vi "Read.vi"(8 "error in (no error)":errorcluster, 9 "timeout ms (5000)":i32=5000, 11 "WebSocket Connection in":refnum<k5>) -> (0 "error out":errorcluster, 1 "Opcode":T1=1 items=["Cont. Frame"=0, "Text"=1, "Binary"=2, "Ping"=9, "Pong"=10], 2 "Data":string, 3 "WebSocket Connection out":refnum<k5>, 4 "Finished?":bool)   [LabVIEW 2013, in "WebSockets.lvlib"]
doc: "Reads and decodes an incoming WebSockets message.\n\nOpcode: Opcode for the message.\nData: Contains the WebSockets payload\nFinished?: Determines whether the message is complete for fragmented messages. If false, must continue to read messages (continuation frames with opcode = 0) until Finished? is true."
uses:
  WebSockets.lvlib
  Opcodes.ctl
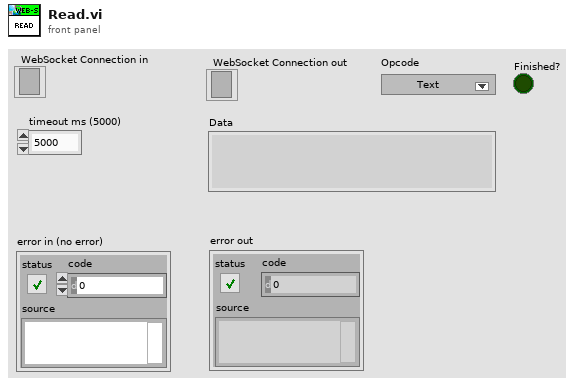
[diagram p1: front panel]
types:
  T1 = typedef "WebSockets.lvlib/Opcodes.ctl" = u8
  T2 = enum16{"big-endian, network order", "native, host order", "little-endian"}
  T3 = enum16{"Standard", "Buffered", "CRLF", "Immediate"}
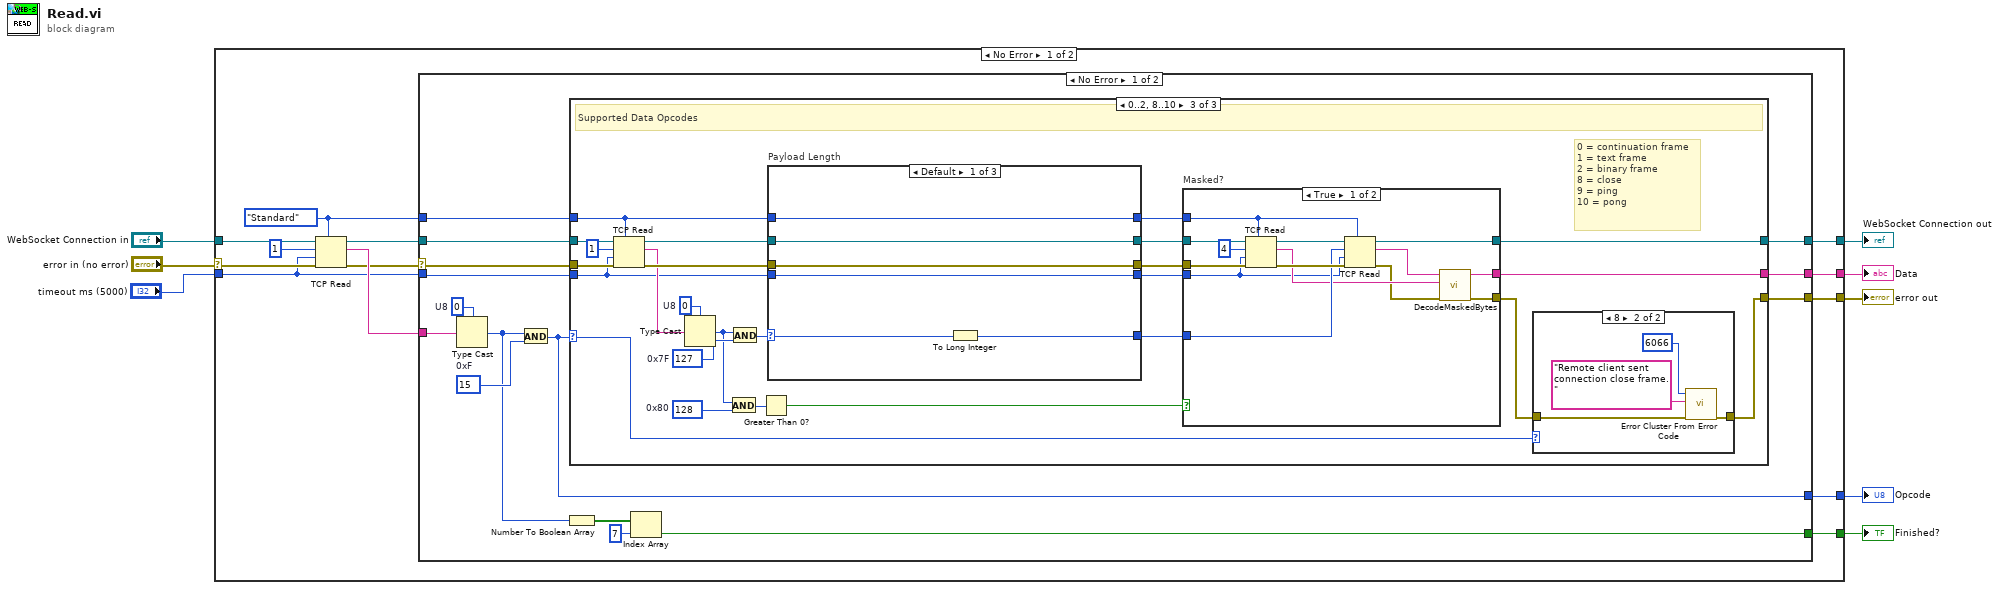
[diagram p0: block diagram]
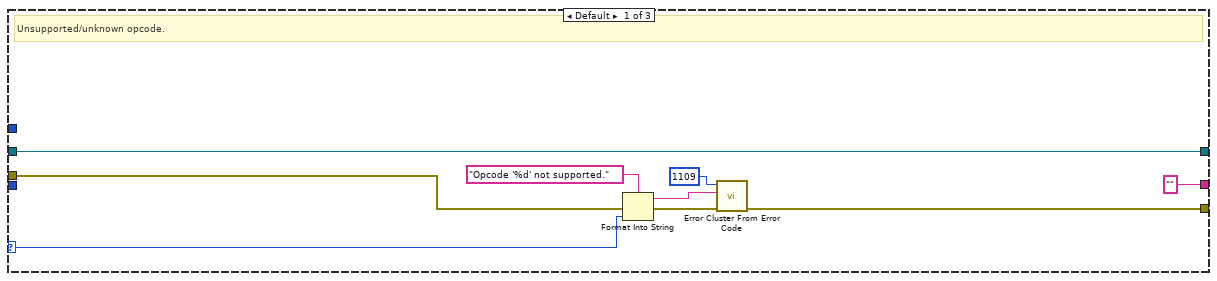
[diagram p2: hidden frame]
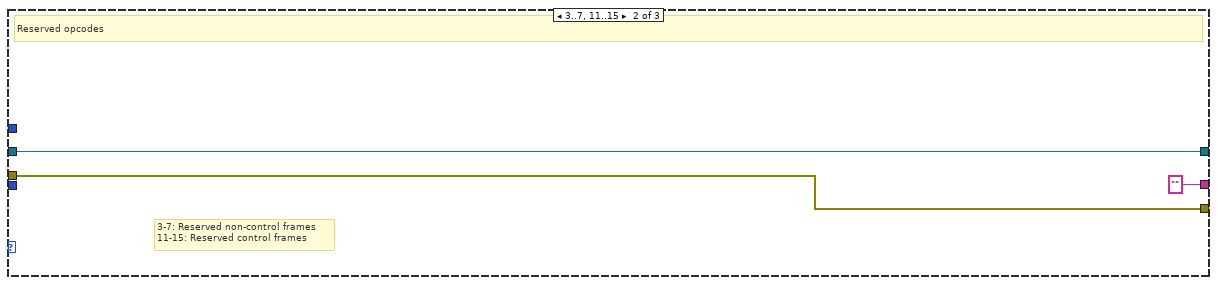
[diagram p3: hidden frame]
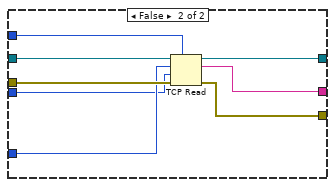
[diagram p5: hidden frame]
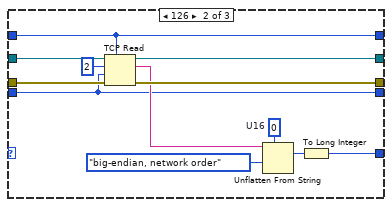
[diagram p6: hidden frame]
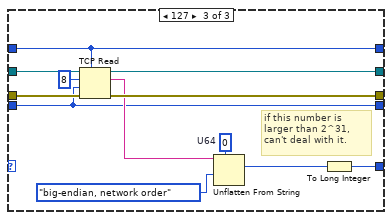
[diagram p7: hidden frame]
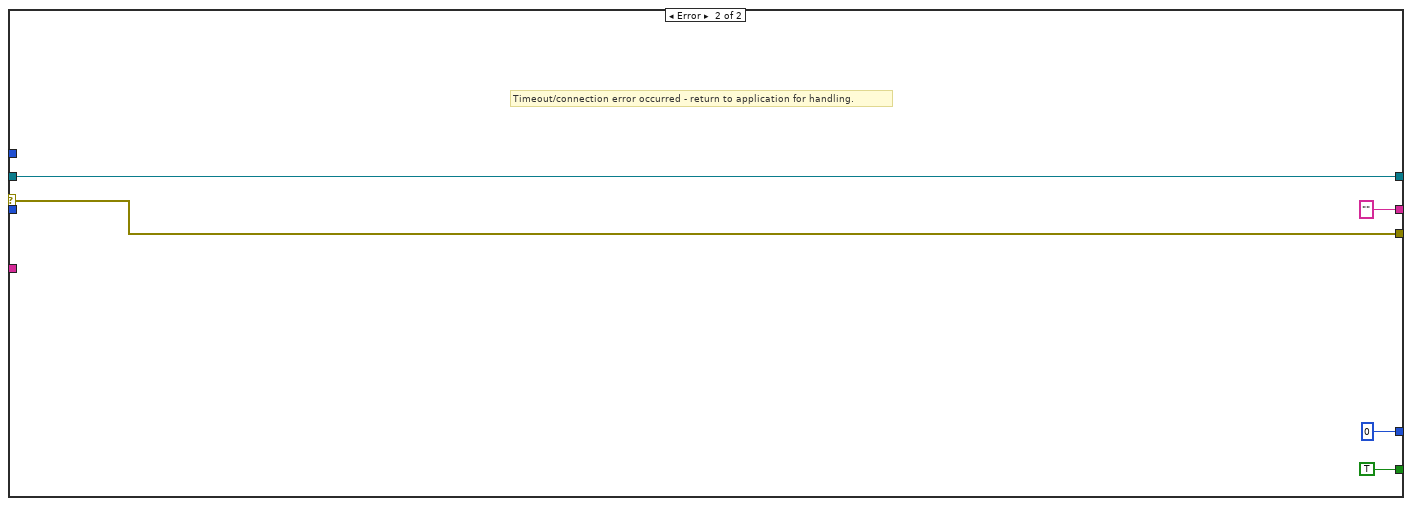
[diagram p8: hidden frame]
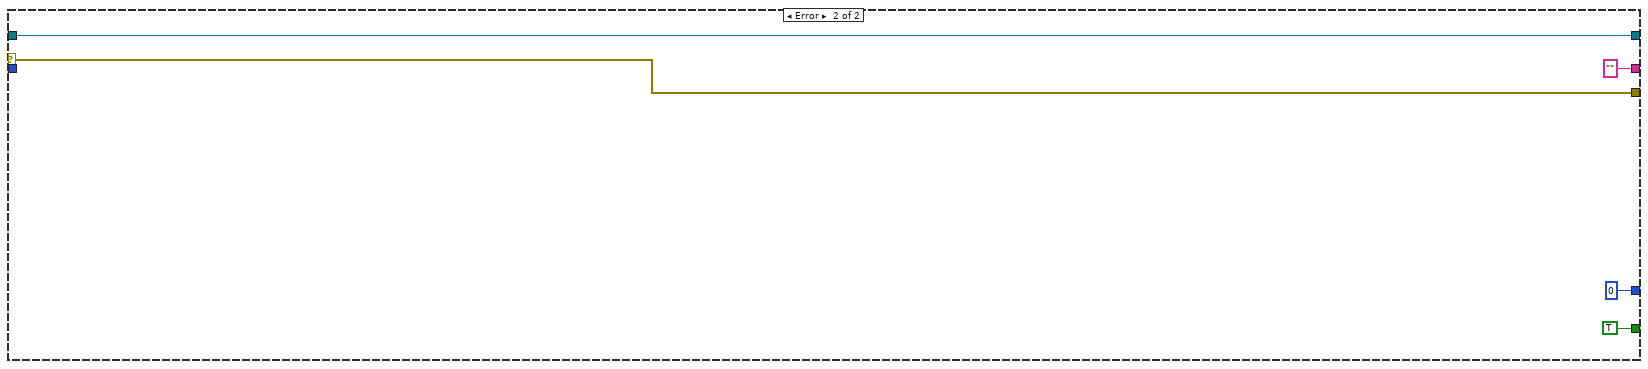
[diagram p9: hidden frame]
diagram:
  n1 = case shown="No Error" "error in (no error)" {
    selector: "error in (no error)" -> [w15 w140]
    tunnel: "WebSocket Connection in" -> [w21 w139]
    tunnel: [w16 w139] -> w7
    tunnel: [w14 "" ("data out")] -> w6
    tunnel: [w13 w140] -> w4
    tunnel: "timeout ms (5000)" -> [w9 _]
    tunnel: [w11 u8 0] -> w1
    tunnel: [w10 TRUE] -> w2
    frame No Error {
      w17 = T3."Standard" ("mode (standard)")
      n2 = TCP Read(connection ID=w21, bytes to read=1, error in (no error)=w15, 7:w17, 9:w9) -> (connection ID out=w18:refnum<k5>, data out=w19:string, error out=w12:errorcluster)
      n3 = case shown="No Error" w12 {
        selector: w12 -> [w31 w133]
        tunnel: w19 -> [w30 _]
        tunnel: w18 -> [w36 w135]
        tunnel: w17 -> [w35 _]
        tunnel: [w34 w135] -> w16
        tunnel: [w33 "" ("Decoded Data")] -> w14
        tunnel: [w32 w133] -> w13
        tunnel: [w27 u8 0] -> w11
        tunnel: [w24 TRUE] -> w10
        tunnel: w9 -> [w23 _]
        frame No Error {
          w28 = u8 15  # 0xF
          w29 = u8 0  # U8
          n4 = Type Cast(type=w29, x=w30) -> (*(type *) &x=w26:u8)
          n5 = And(x=w26, y=w28) -> (x .and. y?=w27:u8)
          n6 = Number To Boolean Array(number=w26) -> (Boolean array=w25:bool[])
          n7 = case shown="0..2, 8..10" w27 {
            selector: w27 -> [w38 _ w53]
            tunnel: w36 -> [w45 w47 w65]
            tunnel: w35 -> [_ _ w63]
            tunnel: [w45 w47 w73] -> w34
            tunnel: ["" ("Decoded Data") "" ("Decoded Data") w66] -> w33
            tunnel: [w43 w48 w51] -> w32
            tunnel: w31 -> [w42 w48 w61]
            tunnel: w23 -> [_ _ w49]
            frame Default {
              # "Unsupported/unknown opcode."
              n8 = Format Into String(format string="Opcode '%d' not supported.", error in=w42, w38) -> (resulting string=w40:string, error out=w41:errorcluster)  [unwired: 1 in]
              n9 = call <vilib>:"Error Cluster From Error Code.vi"("error in (no error)"=w41, "error message (\"\")"=w40, "error code (0)"=1109) -> ("error out"=w43:errorcluster)  [unwired: 6 in]
            }
            frame 3..7, 11..15 {
              # "3-7: Reserved non-control frames\n11-15: Reserved control frames"
              # "Reserved opcodes"
            }
            frame 0..2, 8..10 {
              w57 = u8 128  # 0x80
              w58 = u8 0  # U8
              w72 = u8 127  # 0x7F
              # "0 = continuation frame\n1 = text frame\n2 = binary frame\n8 = close\n9 = ping\n10 = pong"
              # "Supported Data Opcodes"
              n10 = TCP Read(connection ID=w65, bytes to read=1, error in (no error)=w61, 7:w63, 9:w49) -> (connection ID out=w64:refnum<k5>, data out=w59:string, error out=w60:errorcluster)
              n11 = Type Cast(type=w58, x=w59) -> (*(type *) &x=w56:u8)
              n12 = And(x=w56, y=w57) -> (x .and. y?=w55:u8)
              n13 = And(x=w56, y=w72) -> (x .and. y?=w71:u8)
              n14 = Greater Than 0?(x=w55) -> (x > 0?=w54:bool)
              n15 = case "Payload Length" shown="Default" w71 {
                selector: w71 -> [w105 _ _]
                tunnel: w64 -> [w106 w118 w129]
                tunnel: [w106 w117 w128] -> w70
                tunnel: w63 -> [w103 w115 w124]
                tunnel: [w104 w108 w127] -> w67
                tunnel: [w103 w115 w124] -> w69
                tunnel: [w102 w114 w126] -> w68
                tunnel: w60 -> [w102 w113 w125]
                tunnel: w49 -> [w101 w107 w119]
                tunnel: [w101 w107 w119] -> w50
                frame Default {
                  n16 = To Long Integer(number=w105) -> (32bit integer=w104:i32)
                }
                frame 126 {
                  w112 = u16 0  # U16
                  n17 = TCP Read(connection ID=w118, bytes to read=2, error in (no error)=w113, 7:w115, 9:w107) -> (connection ID out=w117:refnum<k5>, data out=w110:string, error out=w114:errorcluster)
                  n18 = Unflatten From String(type=w112, binary string=w110, byte order (0:big-endian, network order)=T2."big-endian, network order") -> (value=w109:u16)  [unwired: 2 in, 2 out]
                  n19 = To Long Integer(number=w109) -> (32bit integer=w108:i32)
                }
                frame 127 {
                  w123 = u64 0  # U64
                  # "if this number is larger than 2^31, can't deal with it."
                  n20 = TCP Read(connection ID=w129, bytes to read=8, error in (no error)=w125, 7:w124, 9:w119) -> (connection ID out=w128:refnum<k5>, data out=w122:string, error out=w126:errorcluster)
                  n21 = Unflatten From String(type=w123, binary string=w122, byte order (0:big-endian, network order)=T2."big-endian, network order") -> (value=w121:u64)  [unwired: 2 in, 2 out]
                  n22 = To Long Integer(number=w121) -> (32bit integer=w127:i32)
                }
              }
              n23 = case "Masked?" shown="True" w54 {
                tunnel: [w92 w100] -> w73
                tunnel: w70 -> [w91 w99]
                tunnel: w69 -> [w89 w98]
                tunnel: w68 -> [w88 w97]
                tunnel: w67 -> [w85 w96]
                tunnel: [w82 w94] -> w66
                tunnel: [w80 w95] -> w52
                tunnel: w50 -> [w79 w93]
                frame True {
                  n24 = TCP Read(connection ID=w91, bytes to read=4, error in (no error)=w88, 7:w89, 9:w79) -> (connection ID out=w90:refnum<k5>, data out=w84:string, error out=w87:errorcluster)
                  n25 = TCP Read(connection ID=w90, bytes to read=w85, error in (no error)=w87, 7:w89, 9:w79) -> (connection ID out=w92:refnum<k5>, data out=w83:string, error out=w81:errorcluster)
                  n26 = call "DecodeMaskedBytes.vi"("error in (no error)"=w81, "Mask Bytes"=w84, "Encoded Data"=w83) -> ("error out"=w80:errorcluster, "Decoded Data"=w82:string)  [unwired: 7 in]
                }
                frame False {
                  n27 = TCP Read(connection ID=w99, bytes to read=w96, error in (no error)=w97, 7:w98, 9:w93) -> (connection ID out=w100:refnum<k5>, data out=w94:string, error out=w95:errorcluster)
                }
              }
              n28 = case shown="8" w53 {
                tunnel: w52 -> [w74 w76]
                tunnel: [w74 w75] -> w51
                frame Default {
                }
                frame 8 {
                  n29 = call <vilib>:"Error Cluster From Error Code.vi"("error in (no error)"=w76, "error message (\"\")"="Remote client sent connection close frame." ("error message (\"\")"), "error code (0)"=6066) -> ("error out"=w75:errorcluster)  [unwired: 6 in]
                }
              }
            }
          }
          n30 = Index Array(array=w25, index=7) -> (element=w24:bool)
        }
        frame Error {
          # "Timeout/connection error occurred - return to application for handling."
        }
      }
    }
    frame Error {
    }
  }
  "WebSocket Connection out" <- w7
  "Data" <- w6
  "error out" <- w4
  "Finished?" <- w2
  "Opcode" <- w1
